vi "Compile Channel Group Settings.vi"(8 "Channel Type":T1(ring), 9 "Group Name":string, 10 "ChannelSettings":T3, 11 "Group Settings":T2[](array[typedef])) -> (3 "Group Settings":T2[](array[typedef]))   [LabVIEW 2026, in "SystemMonitor Deployment Hooks.lvlib"]
uses:
  SystemMonitor Deployment Hooks.lvlib
  Shared/GroupedChannel.ctl
  Shared/GroupSettings.ctl
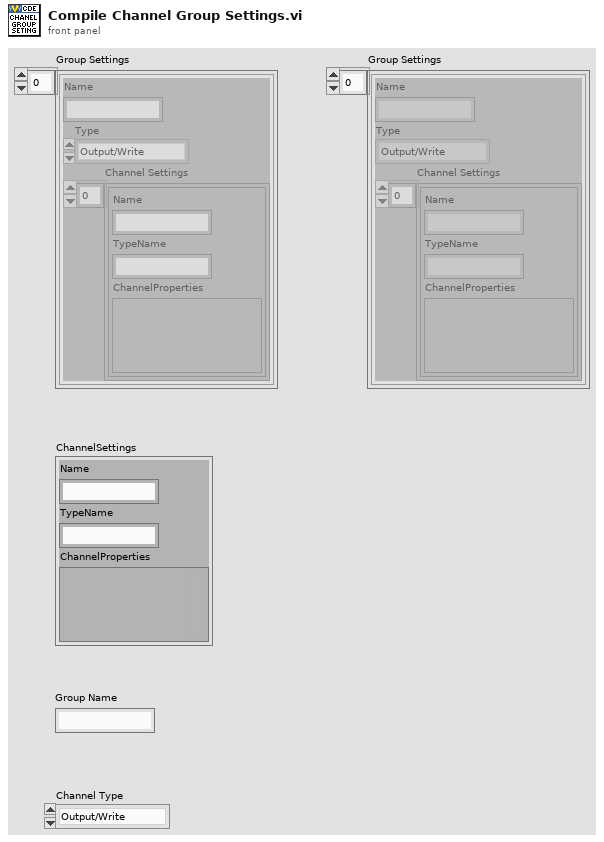
[diagram p1: front panel]
types:
  T1 = enum16{"Output/Write", "Input/Read", "Input/ReadWrite"}
  T2 = typedef "GroupSettings.ctl" = cluster{"Name":string, "Type":enum16{"Output/Write", "Input/Read", "Input/ReadWrite"}, "Channel Settings":T3[]}
  T3 = typedef "GroupedChannel.ctl" = cluster{"Name":string, "TypeName":string, "ChannelProperties":variant}
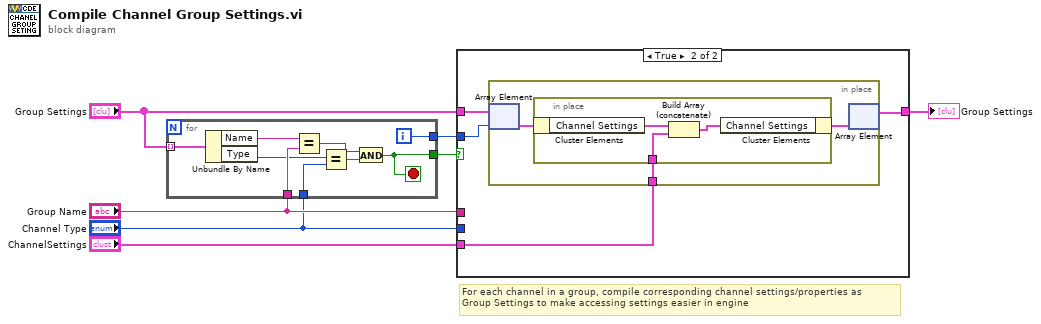
[diagram p0: block diagram]
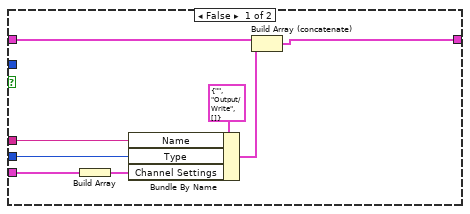
[diagram p2: hidden frame]
diagram:
  # "For each channel in a group, compile corresponding channel settings/properties as\nGroup Settings to make accessing settings easier in engine"
  n1 = for {
    tunnel: "Group Name" -> [w15]
    tunnel: [w12] -> w2
    tunnel: [w13] -> w1
    tunnel: "Group Settings" -> [w14] mode=indexing
    tunnel: "Channel Type" -> [w8]
    i -> [w13]
    stop <- w12 stop-if-true
    n2 = Unbundle By Name(w14) -> ("Name"=w16:string, "Type"=w9:T1)
    n3 = Equal?(x=w16, y=w15) -> (x = y?=w11:bool)
    n4 = Equal?(x=w9, y=w8) -> (x = y?=w10:bool)
    n5 = And(x=w11, y=w10) -> (x .and. y?=w12:bool)
  }
  n6 = case shown="True" w2 {
    tunnel: [w21 w27] -> w6
    tunnel: "Group Settings" -> [w22 w28]
    tunnel: "ChannelSettings" -> [w23 w25]
    tunnel: w1 -> [_ w26]
    tunnel: "Group Name" -> [w24 _]
    tunnel: "Channel Type" -> [w20 _]
    frame False {
      n7 = Build Array(w23) -> (w18:T3[])
      n8 = Bundle By Name(cluster=T2 {"Name"="", "Type"=enum."Output/Write", "Channel Settings"=[]} ("GroupSettings"), "Name"=w24, "Type"=w20, "Channel Settings"=w18) -> (w17:T2)
      n9 = Build Array (concatenate)(w22, w17) -> (w21:T2[])
    }
    frame True {
      n10 = in-place {
        in-place-border: w25 -> [w29]
        n11 = in-place-array #1(w28, w26) -> (w31:T2)
        n12 = in-place {
          in-place-border: w29 -> [w33]
          n13 = in-place-cluster #2(w31) -> ("Channel Settings"=w34:T3[])
          n14 = Build Array (concatenate)(w34, w33) -> (w32:T3[])
          n15 = in-place-cluster #2("Channel Settings"=w32) -> (w30:T2)
        }
        n16 = in-place-array #1(w30) -> (w27:T2[])  [unwired: 1 out]
      }
    }
  }
  "Group Settings" <- w6
